vi "Knob Turn Data.vi"(7 "Switch":T1=enum."Casuals") -> (8 "Switch Message":string)   [LabVIEW 2014]
uses:
  type defs/Encoder Position.ctl
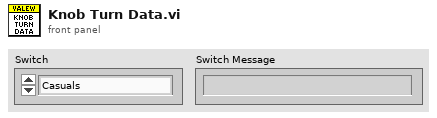
[diagram p1: front panel]
types:
  T1 = typedef "Encoder Position.ctl" = enum16{"Mixed", "Casuals", "Delicates", "Speed Dry", "Jeans", "Time Dry", "Warm Up", "Air Fluff", "Steam Dewrinkle", "Steam Refesh", "Sanitize", "Bulky", "Towels / Sheets", "Cottons", "Clear / Reset"}
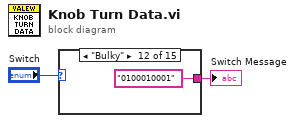
[diagram p0: block diagram]
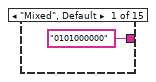
[diagram p2: hidden frame]
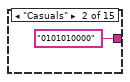
[diagram p3: hidden frame]
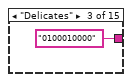
[diagram p4: hidden frame]
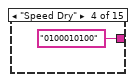
[diagram p5: hidden frame]
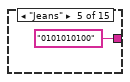
[diagram p6: hidden frame]
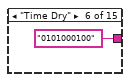
[diagram p7: hidden frame]
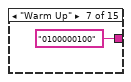
[diagram p8: hidden frame]
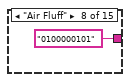
[diagram p9: hidden frame]
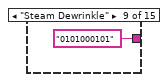
[diagram p10: hidden frame]
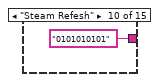
[diagram p11: hidden frame]
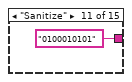
[diagram p12: hidden frame]
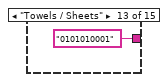
[diagram p13: hidden frame]
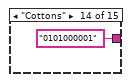
[diagram p14: hidden frame]
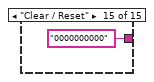
[diagram p15: hidden frame]
diagram:
  n1 = case shown="\"Bulky\"" "Switch" {
    tunnel: ["0101000000" ("Message") "0101010000" ("Message") "0100010000" ("Message") "0100010100" ("Message") "0101010100" ("Message") "0101000100" ("Message") "0100000100" ("Message") "0100000101" ("Message") "0101000101" ("Message") "0101010101" ("Message") "0100010101" ("Message") "0100010001" ("Message") "0101010001" ("Message") "0101000001" ("Message") "0000000000" ("Message")] -> w1
    frame "Mixed", Default {
    }
    frame "Casuals" {
    }
    frame "Delicates" {
    }
    frame "Speed Dry" {
    }
    frame "Jeans" {
    }
    frame "Time Dry" {
    }
    frame "Warm Up" {
    }
    frame "Air Fluff" {
    }
    frame "Steam Dewrinkle" {
    }
    frame "Steam Refesh" {
    }
    frame "Sanitize" {
    }
    frame "Bulky" {
    }
    frame "Towels / Sheets" {
    }
    frame "Cottons" {
    }
    frame "Clear / Reset" {
    }
  }
  "Switch Message" <- w1
